vi "Proof Of Concept.vi"() -> ()   [LabVIEW 2018]
uses:
  builds/Light Stack.lvlibp/Custom Controls/Light Select.ctl
  builds/Light Stack.lvlibp/Custom Controls/Light Mode.ctl
  builds/PLC.lvlibp/PLC.lvclass
  builds/Light Stack.lvlibp
panel:
  in  "State":T1
  in  "Light Select":T2
  out "Output State":bool[](array[boolean])
  out "Inputs":bool[](array[boolean])
  in  "Write":bool
  in  "Output Select":i32
  in  "Value":bool
  in  "stop":bool
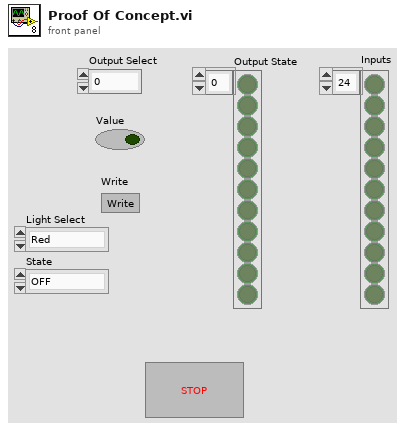
[diagram p1: front panel]
types:
  T1 = typedef "Light Stack.lvlibp/Light Mode.ctl" = enum16{"OFF", "ON", "BLINK"}
  T2 = typedef "Light Stack.lvlibp/Light Select.ctl" = enum16{"Red", "Amber", "Green", "Blue"}
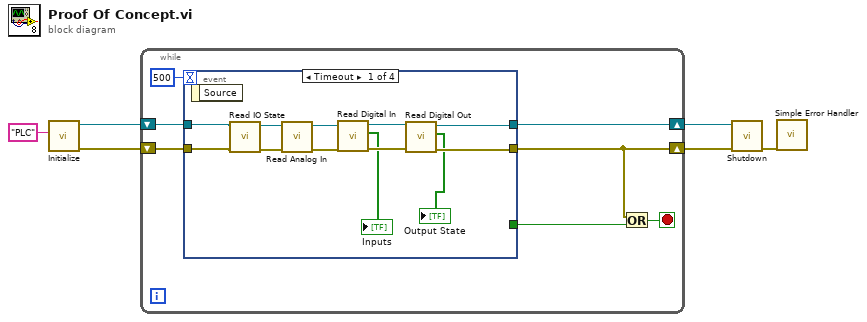
[diagram p0: block diagram]
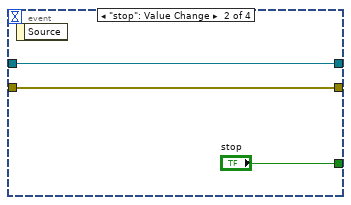
[diagram p2: hidden frame]
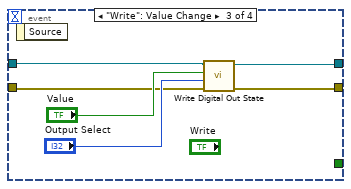
[diagram p3: hidden frame]
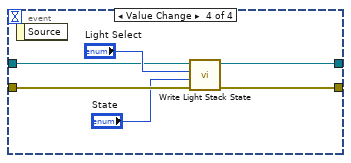
[diagram p4: hidden frame]
diagram:
  n1 = call "Initialize.vi"("Device"="PLC" ("Device Name")) -> ("error out"=w5:errorcluster, "PLC out"=w6:refnum<class "PLC.lvclass">)  [unwired: 9 in]
  n2 = while {
    shift-right: [w10] -> w2
    shift-left: w6 -> [w12]
    shift-right: [w8] -> w3
    shift-left: w5 -> [w11]
    stop <- w7 stop-if-true
    n3 = event shown="[0] Timeout" {
      selector: _ -> [_ _ _ _]
      dyn-events: _ -> [_ _ _ _]
      timeout: 500 -> [_ _ _ _]
      tunnel: w12 -> [w24 w28 w34 w39]
      tunnel: w11 -> [w25 w27 w29 w36]
      tunnel: [w16 w28 w33 w38] -> w10
      tunnel: [w17 w27 w32 w37] -> w8
      tunnel: [_ "stop" _ _] -> w9
      event Timeout {
        n4 = event-data() -> ()  [unwired: 1 in, 1 out]
        n5 = call "Read IO State.vi"("error in"=w25, "PLC in"=w24) -> ("error out"=w22:errorcluster, "PLC out"=w23:refnum<class "PLC.lvclass">)  [unwired: 8 in]
        n6 = call "Read Analog In.vi"("error in"=w22, "PLC in"=w23) -> ("error out"=w21:errorcluster, "PLC out"=w20:refnum<class "PLC.lvclass">)  [unwired: 7 in, 1 out]
        n7 = call "Read Digital In.vi"("error in"=w21, "PLC in"=w20) -> ("error out"=w18:errorcluster, "Digital In"=→"Inputs":bool[], "PLC out"=w19:refnum<class "PLC.lvclass">)  [unwired: 7 in]
        n8 = call "Read Digital Out.vi"("error in"=w18, "PLC in"=w19) -> ("error out"=w17:errorcluster, "Digital Out"=→"Output State":bool[], "PLC out"=w16:refnum<class "PLC.lvclass">)  [unwired: 7 in]
      }
      event "stop": Value Change {
        n9 = event-data() -> ()  [unwired: 1 in, 1 out]
      }
      event "Write": Value Change {
        n10 = event-data() -> ()  [unwired: 1 in, 1 out]
        n11 = call "Write Digital Out State.vi"("error in"=w29, "Selection"="Output Select", "Value"="Value", "PLC in"=w34) -> ("error out"=w32:errorcluster, "PLC out"=w33:refnum<class "PLC.lvclass">)  [unwired: 6 in]
      }
      event Value Change {
        n12 = event-data() -> ()  [unwired: 1 in, 1 out]
        n13 = call "Write Light Stack State.vi"("error in"=w36, "State"="State", "Light Select"="Light Select", "PLC in"=w39) -> ("error out"=w37:errorcluster, "PLC out"=w38:refnum<class "PLC.lvclass">)  [unwired: 6 in]
      }
    }
    n14 = Or(x=w8, y=w9) -> (x .or. y?=w7:bool)
  }
  n15 = call "Shutdown.vi"("error in"=w3, "PLC in"=w2) -> ("error out"=w1:errorcluster)  [unwired: 8 in, 1 out]
  n16 = call <vilib>:"Simple Error Handler.vi"("error in (no error)"=w1) -> ()  [unwired: 4 in, 5 out]
